vi "LIA PLL Simulation.vi"() -> ()   [LabVIEW 2017]
uses:
  <instrlib>/_niInstr/Data Trigger/v1/Shared/Public/Edge Configuration FXP(+-,18,1).ctl
  <instrlib>/_niInstr/Data Trigger/v1/Shared/Public/Edge Configuration Trigger Slope.ctl
  <instrlib>/_niInstr/DSP/v1/Shared/Public/IQ Data.ctl
  <instrlib>/_niInstr/DSP/v1/FPGA/Public/Sub VIs/Frequency Shift/Frequency Shift - 1 spc.vi
  <instrlib>/_niInstr/DSP/v1/Xnodes/Public/Frequency Shift/niInstr DSP v1 Frequency Shift FPGA.xnode
  <instrlib>/_niInstr/DSP/v1/Shared/niInstr DSP v1 Shared.lvlib
  <instrlib>/_niInstr/DSP/v1/FPGA/niInstr DSP v1 FPGA.lvlib
  <instrlib>/_niInstr/Data Trigger/v1/Shared/niInstr Data Trigger v1 Shared.lvlib
panel:
  out "progress":dbl(slide) scale=0.0..1.0
  out "Lock-In Source":dbl(graph)
  out "PLL Source":dbl(graph)
  out "Q":dbl(graph)
  out "I":dbl(graph)
  in  "lock-in.reset":bool
  in  "lock-in.enable":bool
  out "VCO":fxp<+/-,48,0>
  in  "stop":bool
  out "VCO":dbl(graph)
  in  "wait ms":u32=5
  in  "pll.arm":bool
  in  "pll.m":i8=-20
  in  "pll.q":fxp<+,48,0>=0.5000000000000071
  in  "pll.config":T1={"highLevel"=0.25, "lowLevel"=0.0, "trigger slope"=enum."Positive"}
  in  "pll.reset":bool
  in  "file path":path=path "C:/Users/Admin/Desktop/LIA/ADC Samples/Log Files/5783 Digital PLL Capture - 1 MHz Sine.tdms"
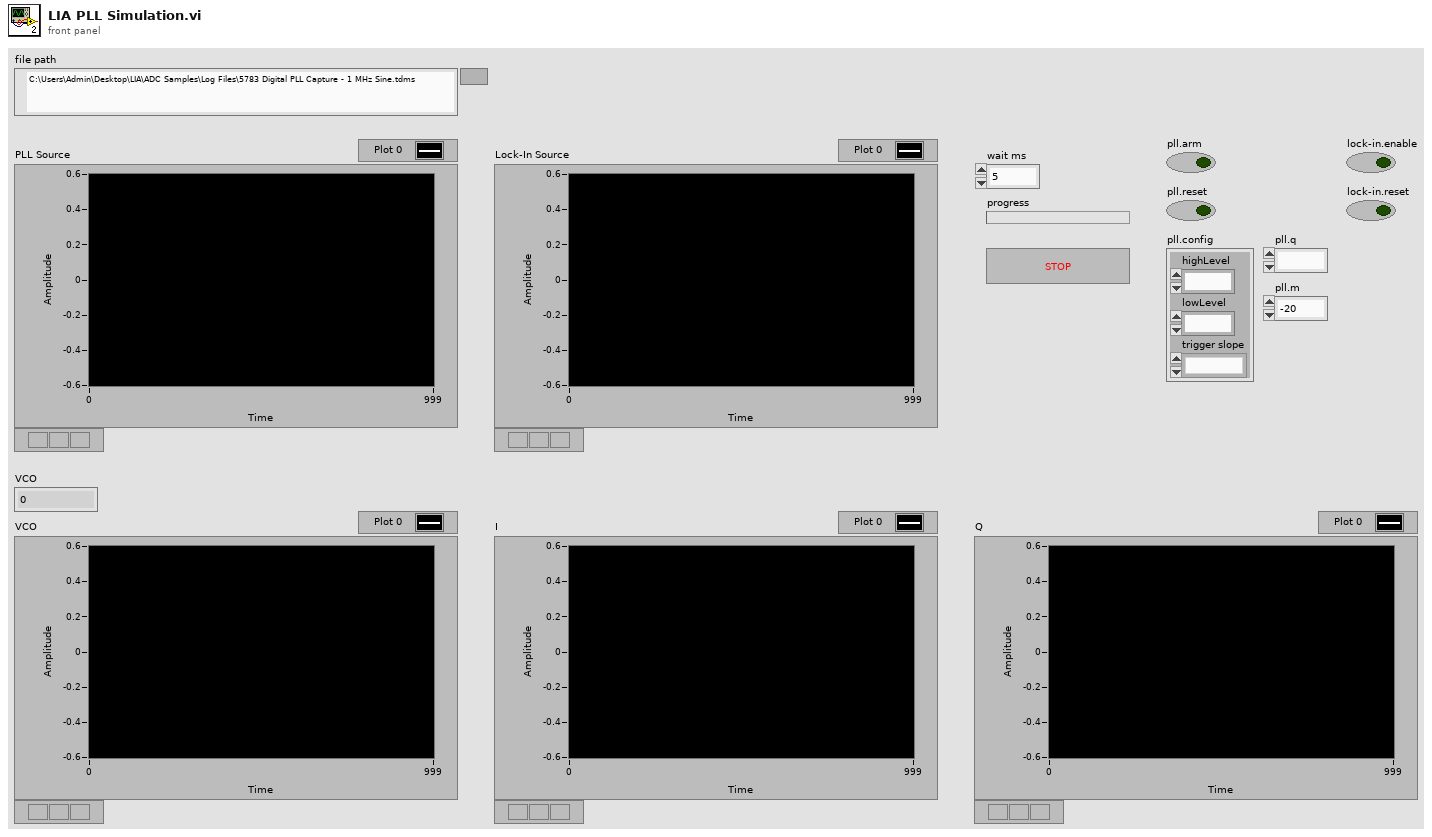
[diagram p1: front panel]
types:
  T1 = typedef "niInstr Data Trigger v1 Shared.lvlib/Edge Configuration FXP(+-,18,1).ctl" = cluster{"highLevel":fxp<+/-,18,1>, "lowLevel":fxp<+/-,18,1>, "trigger slope":T2}
  T2 = typedef "niInstr Data Trigger v1 Shared.lvlib/Edge Configuration Trigger Slope.ctl" = enum8{"Positive", "Negative"}
  T3 = typedef "niInstr DSP v1 Shared.lvlib/IQ Data.ctl" = cluster{"I":fxp<+/-,18,1>, "Q":fxp<+/-,18,1>, "overflow":bool}
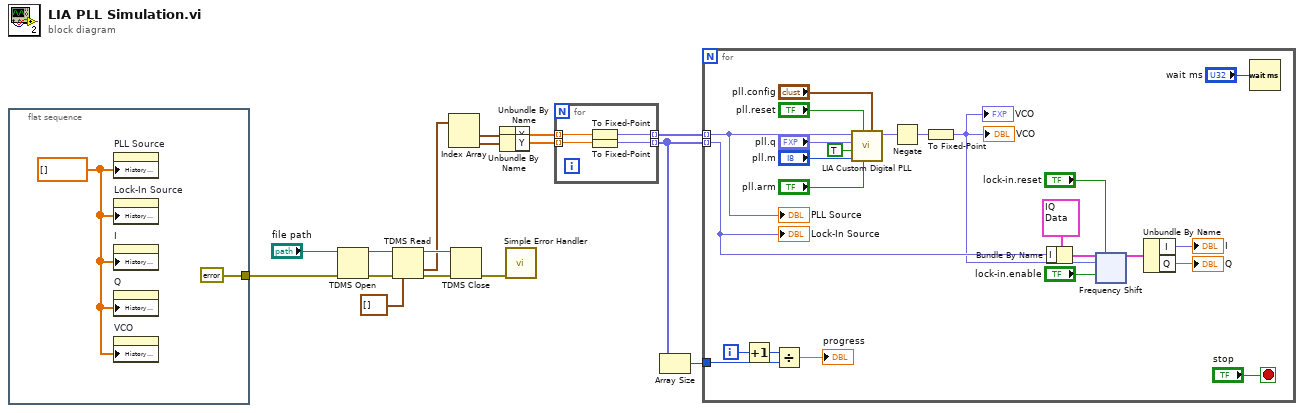
[diagram p0: block diagram]
diagram:
  n1 = flat-sequence {
    tunnel: [errorcluster {"status"=FALSE, "code"=0, "source"=""} ("error constant")] -> w1
    frame #0 {
      w18 = dbl[] [] ("History Data")
      n2 = property on="PLL Source" class="WFChart (strict)"("History Data"=w18) -> ()  [unwired: 2 in, 2 out]
      n3 = property on="Lock-In Source" class="WFChart (strict)"("History Data"=w18) -> ()  [unwired: 2 in, 2 out]
      n4 = property on="I" class="WFChart (strict)"("History Data"=w18) -> ()  [unwired: 2 in, 2 out]
      n5 = property on="Q" class="WFChart (strict)"("History Data"=w18) -> ()  [unwired: 2 in, 2 out]
      n6 = property on="VCO" class="WFChart (strict)"("History Data"=w18) -> ()  [unwired: 2 in, 2 out]
    }
  }
  n7 = TDMS Open(8:w1, 11:"file path") -> (0:w14:errorcluster, 3:w15:refnum<k34>)  [unwired: 5 in]
  n8 = TDMS Read(0:w15, 11:w14, 12:waveform(dbl)[] []) -> (4:w12:refnum<k34>, 10:w10:waveform(dbl)[], 15:w11:errorcluster)  [unwired: 5 in, 3 out]
  n9 = Index Array(array=w10) -> (element #1=w9:waveform(dbl), element #2=w6:waveform(dbl))  [unwired: 2 in]
  n10 = TDMS Close(8:w11, 11:w12) -> (0:w4:errorcluster)  [unwired: 1 out]
  n11 = Unbundle By Name(w9) -> ("Y"=w8:dbl[])
  n12 = Unbundle By Name(w6) -> ("Y"=w7:dbl[])
  n13 = call <vilib>:"Simple Error Handler.vi"("error in (no error)"=w4) -> ()  [unwired: 4 in, 5 out]
  n14 = for {
    tunnel: w8 -> [w22] mode=indexing
    tunnel: [w21] -> w5 mode=indexing
    tunnel: w7 -> [w20] mode=indexing
    tunnel: [w19] -> w3 mode=indexing
    n15 = To Fixed-Point(number=w22) -> (fixed-point=w21:fxp<+/-,18,1>)  [unwired: 1 in]
    n16 = To Fixed-Point(number=w20) -> (fixed-point=w19:fxp<+/-,18,1>)  [unwired: 1 in]
  }
  n17 = Array Size(array=w3) -> (size(s)=w2:i32)
  n18 = for {
    tunnel: w5 -> [w24] mode=indexing
    tunnel: w3 -> [w25] mode=indexing
    tunnel: w2 -> [w29]
    i -> [w27]
    stop <- "stop" stop-if-true
    n19 = Increment(x=w27) -> (x+1=w28:i32)
    n20 = Divide(x=w28, y=w29) -> (x/y=→"progress":dbl)
    n21 = call "LIA Custom Digital PLL.vi"("configuration"="pll.config", "arm"="pll.arm", "reset"="pll.reset", "m"="pll.m", "input valid"=TRUE, "q"="pll.q", "I"=w24) -> ("frequency shift"=w40:fxp<+/-,48,0>)  [unwired: 1 in, 3 out]
    n22 = Negate(x=w40) -> (-x=w35:fxp<+/-,49,1>)
    n23 = To Fixed-Point(number=w35) -> (fixed-point=w23:fxp<+/-,48,0>)  [unwired: 1 in]
    "VCO" <- w23
    "VCO" <- w23
    n24 = Bundle By Name(cluster=T3 {"I"=0.0, "Q"=0.0, "overflow"=FALSE} ("data"), "I"=w25) -> (w36:T3)
    n25 = xnode "Frequency Shift"("data in"=w36, "reset"="lock-in.reset", "frequency shift"=w23, "input valid"="lock-in.enable") -> ("data out"=w32:T3)  [unwired: 2 in, 2 out]
    n26 = Unbundle By Name(w32) -> ("I"=→"I":fxp<+/-,18,1>, "Q"=→"Q":fxp<+/-,18,1>)
    n27 = Wait (ms)(milliseconds to wait="wait ms") -> ()  [unwired: 1 out]
    "PLL Source" <- w24
    "Lock-In Source" <- w25
  }
